vi "msgsBuilder_MasterMessage.vi"(7 "liftState":i32, 9 "position":cluster{"x":dbl, "y":dbl, "z":dbl}) -> (4 "msg out":string)   [LabVIEW 2016]
uses:
  builds/UnicornMain/UnicornRIO1/ROS for LabVIEW/home/lvuser/natinst/bin/user.lib/ROS for LabVIEW Software/ROS/MessageBuilding/std_msgs/subs/i32Scalar.vi
  builds/UnicornMain/UnicornRIO1/ROS for LabVIEW/home/lvuser/natinst/bin/user.lib/ROS for LabVIEW Software/ROS/MessageBuilding/std_msgs/subs/float32Array.vi
panel:
  in  "Array":dbl[](array[numeric])
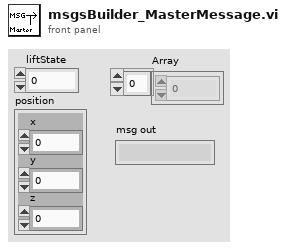
[diagram p1: front panel]
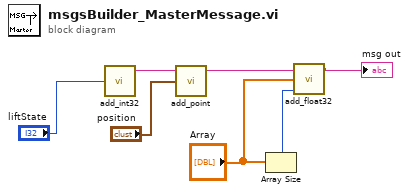
[diagram p0: block diagram]
diagram:
  n1 = call-poly "add_int32.vi"("Numeric"="liftState") -> ("msg out"=w7:string)  [unwired: 4 in]
  n2 = call "add_point.vi"("Point"="position", "msg in"=w7) -> ("msg out"=w2:string)  [unwired: 3 in]
  n3 = Array Size(array="Array") -> (size(s)=w5:i32)
  n4 = call-poly "add_float32.vi"("Array Length"=w5, "Array"="Array", "msg in"=w2) -> ("msg out"=→"msg out":string)  [unwired: 2 in]
